vi "Insert Panel into SubPanel.vi"(8 "error in (no error)":errorcluster, 9 "SubPanel":refnum<vi>, 10 "Panel In":refnum<class "Panel.lvclass">, 11 "Manager in":refnum<class "Manager.lvclass">) -> (0 "error out":errorcluster, 2 "Panel":refnum<class "Panel.lvclass">, 3 "Manager out":refnum<class "Manager.lvclass">)   [LabVIEW 2020, in "OOPanel.lvlib" / "Manager.lvclass"]
uses:
  Manager.lvclass
  Panel/Panel.lvclass
  Panel/Visibility State.ctl
  Manager.lvclass/Manager.ctl
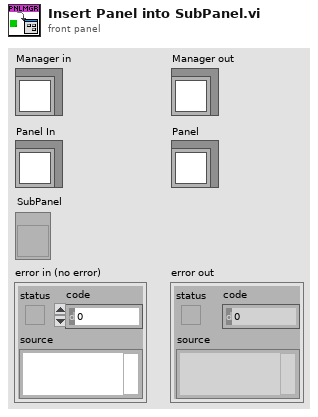
[diagram p1: front panel]
types:
  T1 = typedef "OOPanel.lvlib/Panel.lvclass/Visibility State.ctl" = enum16{"Idle", "Closed", "Hidden", "Visible", "Subpanel"}
  T2 = typedef "OOPanel.lvlib/Manager.lvclass/Ref Data.ctl" = cluster{"SubPanel Map":T3, "Panels":refnum<class "Panel.lvclass">[]}
  T3 = typedef "OOPanel.lvlib/Manager.lvclass/SubPanel Map.ctl" = cluster{"SubPanels":refnum<vi>[], "Panels":refnum<class "Panel.lvclass">[]}
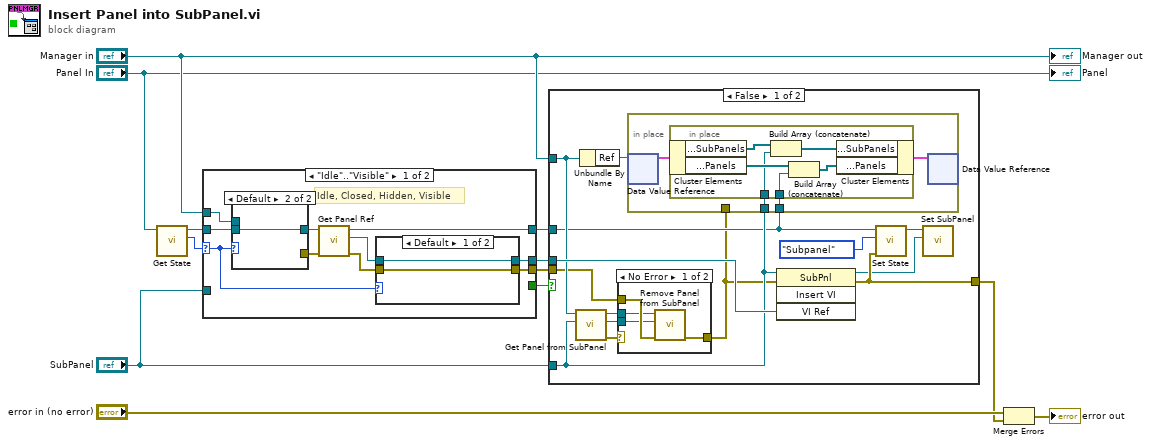
[diagram p0: block diagram]
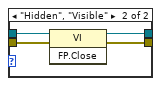
[diagram p2: hidden frame]
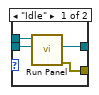
[diagram p3: hidden frame]
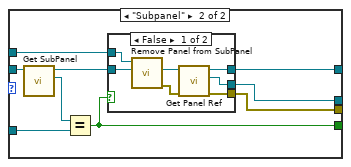
[diagram p4: hidden frame]
diagram:
  n1 = call "Get State.vi"("Panel in"="Panel In") -> ("State"=w10:T1, "Panel out"=w11:refnum<class "Panel.lvclass">)  [unwired: 8 in, 1 out]
  n2 = case shown="\"Idle\"..\"Visible\"" w10 {
    selector: w10 -> [w13 _]
    tunnel: w11 -> [w22 w38]
    tunnel: "Manager in" -> [w21 w42]
    tunnel: [w16 w39] -> w2
    tunnel: [w15 w40] -> w8
    tunnel: [w14 w41] -> w9
    tunnel: "SubPanel" -> [_ w37]
    tunnel: [_ w35] -> w4
    frame "Idle".."Visible" {
      # "Idle, Closed, Hidden, Visible"
      n3 = case shown="Default" w13 {
        tunnel: w22 -> [w32 w33]
        tunnel: w21 -> [w31 _]
        tunnel: [w30 w33] -> w20
        tunnel: [w29 _] -> w19
        frame "Idle" {
          n4 = call "Run Panel.vi"("Panel In"=w32, "Manager in"=w31) -> ("error out"=w29:errorcluster, "Panel"=w30:refnum<class "Panel.lvclass">)  [unwired: 7 in, 1 out]
        }
        frame Default {
        }
      }
      n5 = call "Get Panel Ref.vi"("error in (no error)"=w19, "Panel in"=w20) -> ("error out"=w18:errorcluster, "Panel Ref"=w17:refnum<vi>, "Panel out"=w14:refnum<class "Panel.lvclass">)  [unwired: 7 in]
      n6 = case shown="Default" w13 {
        tunnel: w18 -> [w23 w28]
        tunnel: w17 -> [w24 w27]
        tunnel: [w23 w26] -> w16
        tunnel: [w24 w25] -> w15
        frame Default {
        }
        frame "Hidden", "Visible" {
          n7 = invoke class="VI" method="FP.Close"(reference=w27, error in=w28) -> (reference out=w25:refnum<vi>, error out=w26:errorcluster)  [unwired: 1 in, 1 out]
        }
      }
    }
    frame "Subpanel" {
      n8 = call "Get SubPanel.vi"("Panel in"=w38) -> ("SubPanel"=w36:refnum<vi>, "Panel out"=w34:refnum<class "Panel.lvclass">)  [unwired: 8 in, 1 out]
      n9 = Equal?(x=w36, y=w37) -> (x = y?=w35:bool)
      n10 = case shown="False" w35 {
        tunnel: w42 -> [w49 _]
        tunnel: [w47 _] -> w41
        tunnel: [w46 _] -> w40
        tunnel: [w44 _] -> w39
        tunnel: w34 -> [w43 _]
        frame False {
          n11 = call "Remove Panel from SubPanel.vi"("Panel In"=w43, "Manager in"=w49) -> ("error out"=w45:errorcluster, "Panel"=w48:refnum<class "Panel.lvclass">)  [unwired: 7 in, 1 out]
          n12 = call "Get Panel Ref.vi"("error in (no error)"=w45, "Panel in"=w48) -> ("error out"=w44:errorcluster, "Panel Ref"=w46:refnum<vi>, "Panel out"=w47:refnum<class "Panel.lvclass">)  [unwired: 7 in]
        }
        frame True {
        }
      }
    }
  }
  n13 = case shown="False" w4 {
    tunnel: "Manager in" -> [w57 _]
    tunnel: w9 -> [w55 _]
    tunnel: "SubPanel" -> [w58 _]
    tunnel: w8 -> [w59 _]
    tunnel: [w54 _] -> w6
    tunnel: w2 -> [w56 _]
    frame False {
      n14 = call "Get Panel from SubPanel.vi"("SubPanel"=w58, "Manager in"=w57) -> ("error out"=w61:errorcluster, "Panel"=w62:refnum<class "Panel.lvclass">, "Manager out"=w60:refnum<class "Manager.lvclass">)  [unwired: 7 in]
      n15 = Unbundle By Name(w57) -> ("Ref"=w63:refnum<data-value>)
      n16 = case shown="No Error" w61 {
        tunnel: w62 -> [w75 _]
        tunnel: w60 -> [w76 _]
        tunnel: [w74 w78] -> w52
        tunnel: w56 -> [w77 w78]
        frame No Error {
          n17 = call "Remove Panel from SubPanel.vi"("error in (no error)"=w77, "Panel In"=w75, "Manager in"=w76) -> ("error out"=w74:errorcluster)  [unwired: 6 in, 2 out]
        }
        frame Error {
        }
      }
      n18 = in-place {
        in-place-border: w58 -> [w65]
        in-place-border: w55 -> [w64]
        in-place-border: w52 -> [_]
        n19 = in-place-dvr #1(w63) -> (w67:T2)  [unwired: 1 out]
        n20 = in-place {
          in-place-border: w65 -> [w70]
          in-place-border: w64 -> [w69]
          n21 = in-place-cluster #2(w67) -> ("SubPanel Map.SubPanels"=w71:refnum<vi>[], "SubPanel Map.Panels"=w73:refnum<class "Panel.lvclass">[])
          n22 = Build Array (concatenate)(w71, w70) -> (w72:refnum<vi>[])
          n23 = Build Array (concatenate)(w73, w69) -> (w68:refnum<class "Panel.lvclass">[])
          n24 = in-place-cluster #2("SubPanel Map.SubPanels"=w72, "SubPanel Map.Panels"=w68) -> (w66:T2)
        }
        n25 = in-place-dvr #1(w66) -> ()  [unwired: 2 out]
      }
      n26 = invoke class="SubPnl" method="Insert VI"(reference=w58, error in=w52, "VI Ref"=w59) -> (reference out=w50:refnum<vi>, error out=w54:errorcluster)  [unwired: 1 in, 2 out]
      n27 = call "Set State.vi"("error in (no error)"=w54, "State"=Visibility_State."Subpanel", "Panel in"=w55) -> ("Panel out"=w51:refnum<class "Panel.lvclass">)  [unwired: 7 in, 1 out]
      n28 = call "Set SubPanel.vi"("SubPanel"=w50, "Panel in"=w51) -> ()  [unwired: 8 in, 2 out]
    }
    frame True {
    }
  }
  n29 = Merge Errors("error in (no error)", w6) -> (→"error out":errorcluster)
  "Manager out" <- "Manager in"
  "Panel" <- "Panel In"
